vi "Test Boolean.vi"(7 "Name":string="Test Boolean", 10 "Succeed State":T1, 11 "Abs_Boolean.lvclass":refnum<class "Abs_Boolean.lvclass">) -> (3 "abs_Node":refnum<class "abs_Node.lvclass">)   [LabVIEW 2021, in "BT.lvlib"]
uses:
  BT.lvlib
  abs_Node/abs_Node.lvclass
  abs_Test Boolean/Support/Succeed State.ctl
  GitHub/LV_Abstract/Source/Abs_Types/Boolean/Abs_Boolean.lvclass
  C:/Users/Tim/Documents/GitHub/LV_Abstract/Source/Abs_Types/Type/Abs_Type.lvclass
  Test Boolean/Test Boolean.lvclass
  C:/Users/Tim/Documents/LabVIEW/2021/Behaviour Tree/Source/abs_Type Leaf/abs_Type Leaf.lvclass
  C:/Users/Tim/Documents/LabVIEW/2021/Behaviour Tree/Source/abs_Node/abs_Node.lvclass
  abs_Type Leaf/abs_Type Leaf.lvclass/abs_Type Leaf.ctl
  abs_Node/abs_Node.lvclass/abs_Node.ctl
  Test Boolean/Test Boolean.lvclass/Test Boolean.ctl
  abs_Type Leaf/Properties/Write Value Class.vi
  abs_Node/Properties/Write Name.vi
  Test Boolean/Properties/Write Succeed State .vi
  abs_Test Boolean/abs_Test Boolean.lvclass
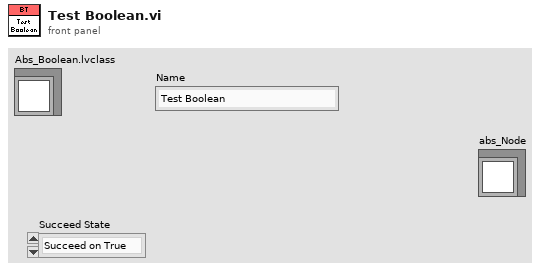
[diagram p1: front panel]
types:
  T1 = typedef "BT.lvlib/abs_Test Boolean.lvclass/Succeed State.ctl" = enum16{"Succeed on True", "Succeed on Fail"}
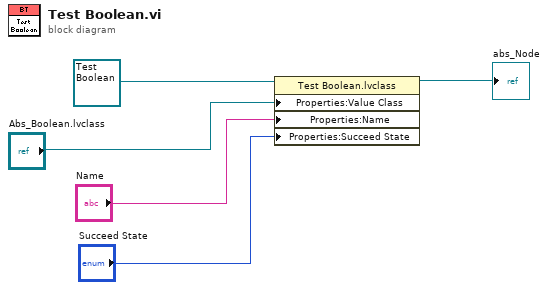
[diagram p0: block diagram]
diagram:
  n1 = property class="Test Boolean.lvclass"(reference=refnum<class "Test Boolean.lvclass"> refnum ("BT.lvlib:Test Boolean.lvclass"), "Properties:Value Class"="Abs_Boolean.lvclass", "Properties:Name"="Name", "Properties:Succeed State "="Succeed State") -> (reference out=→"abs_Node":refnum<class "Test Boolean.lvclass">)  [unwired: 1 in, 1 out]
